vi "UR Script Command.vi"() -> ()   [LabVIEW 2016]
panel:
  in  "exit":bool
  in  "send":bool
  in  "command":string
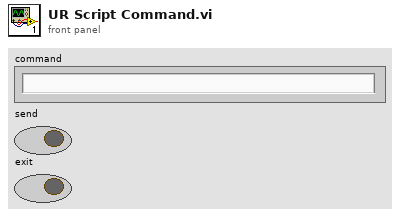
[diagram p1: front panel]
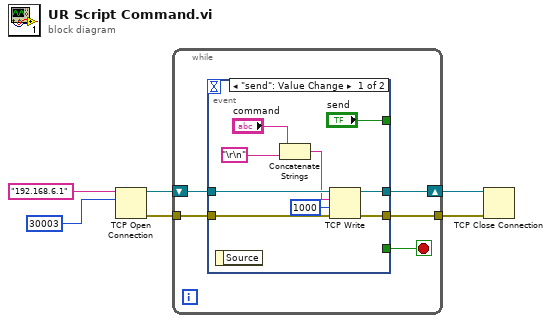
[diagram p0: block diagram]
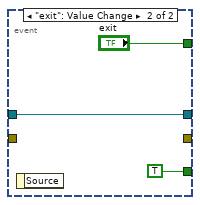
[diagram p2: hidden frame]
diagram:
  n1 = TCP Open Connection(address="192.168.6.1", remote port or service name=u16 30003) -> (connection ID=w4:refnum<k5>, error out=w3:errorcluster)  [unwired: 3 in]
  n2 = while {
    shift-right: [w8] -> w1
    shift-left: w4 -> [w11]
    tunnel: w3 -> [w10]
    tunnel: [w9] -> w2
    stop <- w7 stop-if-true
    n3 = event shown="[0] \"send\": Value Change" {
      selector: _ -> [_ _]
      dyn-events: _ -> [_ _]
      timeout: _ -> [_ _]
      tunnel: w11 -> [w20 w22]
      tunnel: w10 -> [w19 _]
      tunnel: [w18 _] -> w9
      tunnel: [w17 w22] -> w8
      tunnel: ["send" "exit"] -> _
      tunnel: [_ TRUE] -> w7
      event "send": Value Change {
        n4 = event-data() -> ()  [unwired: 1 in, 1 out]
        n5 = Concatenate Strings("command", "\r\n") -> (w14:string)
        n6 = TCP Write(connection ID=w20, data in=w14, error in (no error)=w19, 9:1000 ("timeout ms (25000)")) -> (connection ID out=w17:refnum<k5>, error out=w18:errorcluster)  [unwired: 1 out]
      }
      event "exit": Value Change {
        n7 = event-data() -> ()  [unwired: 1 in, 1 out]
      }
    }
  }
  n8 = TCP Close Connection(connection ID=w1, error in (no error)=w2) -> ()  [unwired: 1 in, 2 out]
